vi "AppPath.vi"() -> (0 "AppPath":path)   [LabVIEW 2020]
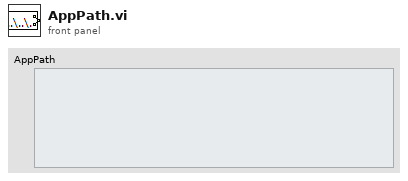
[diagram p1: front panel]
types:
  T1 = enum32{"invalid app kind", "Development System", "Run Time System", "Student Edition", "Embedded LabVIEW", "Evaluation", "Custom"}
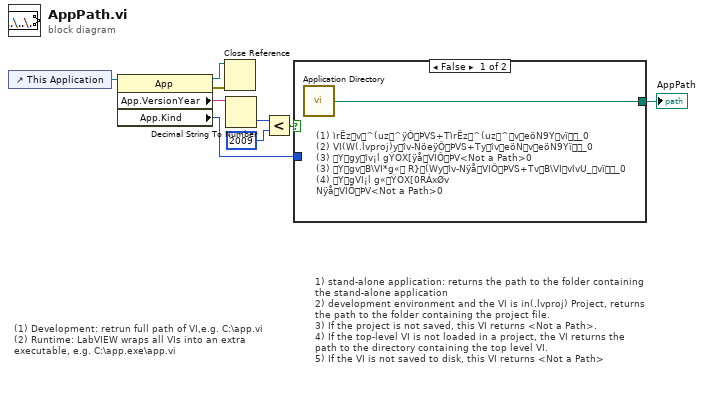
[diagram p0: block diagram]
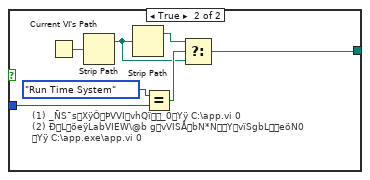
[diagram p2: hidden frame]
diagram:
  # "(1) Development: retrun full path of VI,e.g. C:\\app.vi\n(2) Runtime: LabVIEW wraps all VIs into an extra executable, e.g. C:\\app.exe\\app.vi"
  # "1) stand-alone application: returns the path to the folder containing the stand-alone application\n2) development environment and the VI is in(.lvproj) Project, returns the path to the folder containing the project file.\n3) If the project is not saved, this VI returns <Not a Path>. \n4) If the top-level VI is not loaded in a project, the VI returns the path to the directory containing the top level VI.\n5) If the VI is not saved to disk, this VI returns <Not a Path>"
  n1 = control-ref of="This Application"() -> (w9:refnum<vi>)
  n2 = property class="App"(reference=w9) -> (reference out=w7:refnum<vi>, error out=w8:errorcluster, "App.VersionYear"=w6:string, "App.Kind"=w2:T1)  [unwired: 1 in]
  n3 = Close Reference(reference=w7, error in (no error)=w8) -> ()  [unwired: 1 out]
  n4 = Decimal String To Number(string=w6) -> (number=w5:i32)  [unwired: 2 in, 1 out]
  n5 = Less?(x=w5, y=2009) -> (x < y?=w3:bool)
  n6 = case shown="False" w3 {
    tunnel: w2 -> [_ w16]
    tunnel: [w10 w12] -> w1
    frame False {
      # "(1) ìrËzv^(uz^ÿÔÞVS+TìrËz^(uz^veöN9Yvï_0\n(2) VI(W(.lvproj)yîv-NöeÿÔÞVS+TyîveöNveöN9Yï_0\n(3) Ygyîv¡l\tgÝOX[ÿåVIÔÞV<Not a Path>0\n(3) YgvB\\VI*g« R}(Wyîv-NÿåVIÔÞVS+TvB\\VIvîvU_vï_0\n(4) YgVI¡l\tg«ÝOX[0RÁxØv\nNÿåVIÔÞV<Not a Path>0"
      n7 = call <vilib>:"Application Directory.vi"() -> ("Application Directory"=w10:path)
    }
    frame True {
      # "(1) _ÑS¯sXÿÔÞVVIvhQï_0Yÿ C:\\app.vi 0\n(2) ÐLöeÿLabVIEW\\@b\tgvVISÅbN*NYvïSgbLeöN0\nYÿ C:\\app.exe\\app.vi 0"
      n8 = Current VI's Path() -> (path=w11:path)
      n9 = Strip Path(path=w11) -> (stripped path=w13:path)  [unwired: 1 out]
      n10 = Strip Path(path=w13) -> (stripped path=w14:path)  [unwired: 1 out]
      n11 = Equal?(x=T1."Run Time System" ("Application:Kind"), y=w16) -> (x = y?=w17:bool)
      n12 = Select(t=w14, s=w17, f=w13) -> (s? t:f=w12:path)
    }
  }
  "AppPath" <- w1
